vi "Read configuration.vi"(8 "error in":errorcluster, 11 "TEST EDITOR in":refnum<class "TEST EDITOR.lvclass">) -> (0 "error out":errorcluster, 2 "configuration":refnum<class "NISE_CEF_serializable configuration.lvclass">, 3 "TEST EDITOR out":refnum<class "TEST EDITOR.lvclass">)   [LabVIEW 2013, in "configuration tests.lvlib" / "TEST EDITOR.lvclass"]
uses:
  TEST EDITOR.lvclass
  <vilib>/NI/Configuration Framework/serializable configuration/NISE_CEF_serializable configuration.lvclass
  TEST EDITOR.lvclass/TEST EDITOR.ctl
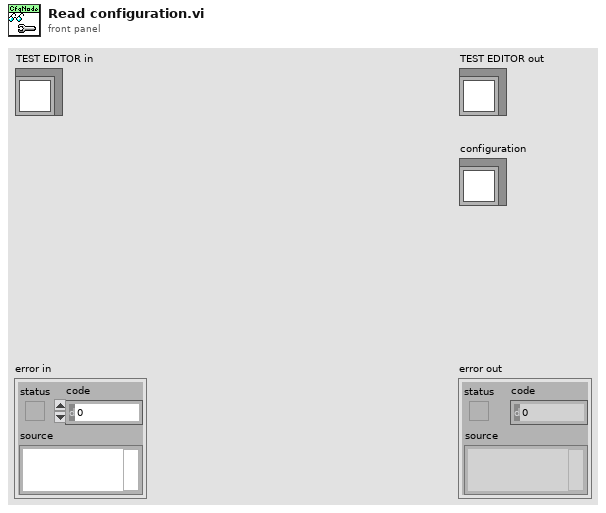
[diagram p1: front panel]
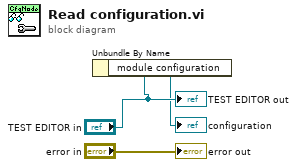
[diagram p0: block diagram]
diagram:
  n1 = Unbundle By Name("TEST EDITOR in") -> ("module configuration"=→"configuration":refnum<class "TEST CONFIGURATION.lvclass">)
  "error out" <- "error in"
  "TEST EDITOR out" <- "TEST EDITOR in"
